vi "ContadorSumaResta.vi"() -> ()   [LabVIEW 2025]
panel:
  out "Numeric":dbl
  in  "stop":bool
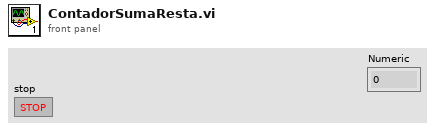
[diagram p1: front panel]
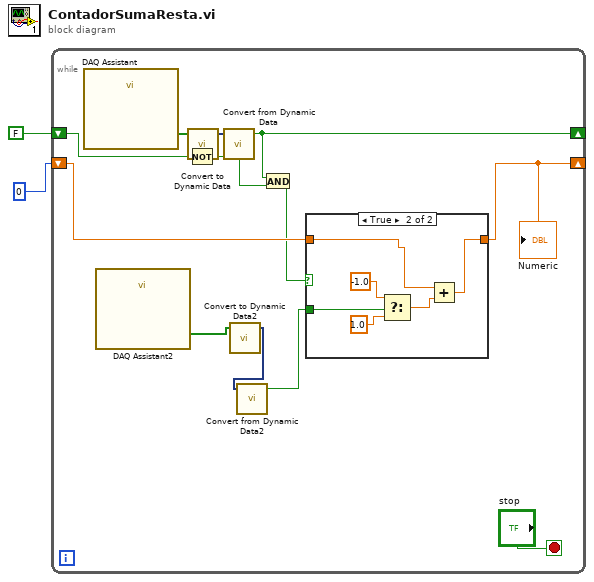
[diagram p0: block diagram]
diagram:
  n1 = while {
    shift-right: [w8] -> _
    shift-left: FALSE -> [w14]
    shift-right: [w3] -> _
    shift-left: 0 -> [w9]
    stop <- "stop" stop-if-true
    n2 = call "DAQ Assistant"() -> ("data"=w12:bool[])  [unwired: 17 in, 2 out]
    n3 = call "DAQ Assistant2"() -> ("data"=w6:bool[])  [unwired: 17 in, 2 out]
    n4 = Not(x=w14) -> (.not. x?=w13:bool)
    n5 = call "Convert to Dynamic Data"("Array"=w12) -> ("Dynamic Data Type"=w11:dynamicdata)  [unwired: 3 in]
    n6 = call "Convert from Dynamic Data"("Dynamic Data Type"=w11) -> ("Scalar"=w8:bool)  [unwired: 3 in]
    n7 = call "Convert to Dynamic Data2"("Array"=w6) -> ("Dynamic Data Type"=w5:dynamicdata)  [unwired: 3 in]
    n8 = call "Convert from Dynamic Data2"("Dynamic Data Type"=w5) -> ("Scalar"=w4:bool)  [unwired: 3 in]
    n9 = And(x=w8, y=w13) -> (x .and. y?=w7:bool)
    n10 = case shown="True" w7 {
      tunnel: w9 -> [w15 w19]
      tunnel: [w15 w17] -> w3
      tunnel: w4 -> [_ w16]
      frame False {
      }
      frame True {
        n11 = Select(t=-1.0, s=w16, f=1.0) -> (s? t:f=w18:dbl)
        n12 = Add(x=w19, y=w18) -> (x+y=w17:dbl)
      }
    }
    "Numeric" <- w3
  }
